vi "Main.vi"() -> ()   [LabVIEW 2019]
doc: "This sample project is built upon the standard state machine template and shows how you could create an application that acquires, analyzes, and presents data. It includes functionality for presenting configuration dialogs, preserving settings between executions, loading and saving data, as well as exporting graph images and text files.\n\nIt is most appropriate for data that is acquired instantly as it does not allow for screen updates mid acquisition nor does it allow for continuous streaming to disk."
uses:
  controls/State.ctl
  controls/Data.ctl
  controls/UI References.ctl
  controls/Graph Data.ctl
  <vilib>/Utility/miscctls.llb/LVAnnotationListTypeDef.ctl
  <vilib>/Utility/miscctls.llb/LVCursorListTypeDef.ctl
  controls/User Specified Data.ctl
  controls/HW Configuration.ctl
  controls/Simulated Signal Type.ctl
  controls/Analysis Configuration.ctl
  controls/New Data Behavior.ctl
  subVIs/Settings Dialog.vi
panel:
  in  "Settings":bool
  in  "Snapshot":bool
  in  "Analyze":bool
  in  "Clear":bool
  in  "Exit":bool
  in  "Acquire":bool
  in  "Export":bool
  in  "Save Data":bool
  in  "Load Data":bool
  out "Graph":waveform(dbl)[](graph)
  out "Status Bar":string
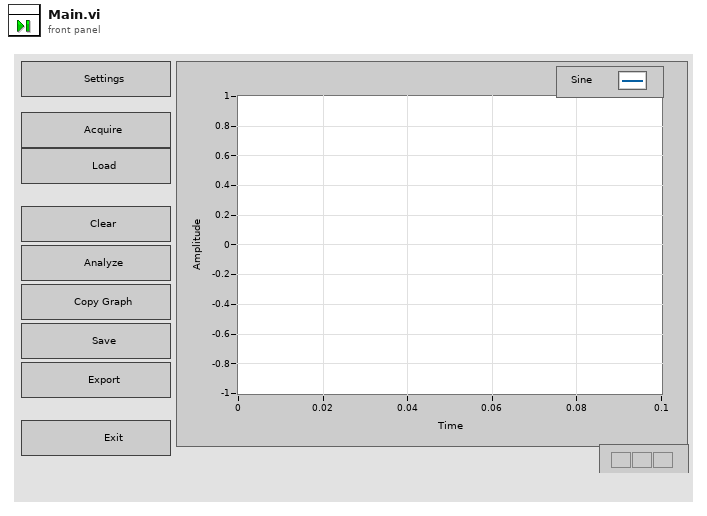
[diagram p1: front panel]
types:
  T1 = typedef "Data.ctl" = cluster{"UI References":T2, "Graph Data":T3, "User Specified":T6}
  T2 = typedef "UI References.ctl" = cluster{"Exit Ref":refnum<vi>, "Save Ref":refnum<vi>, "Open Ref":refnum<vi>, "Export Ref":refnum<vi>, "Acquire Ref":refnum<vi>, "Configure Ref":refnum<vi>, "Graph Ref":refnum<vi>, "Clear Ref":refnum<vi>, "Analyze Ref":refnum<vi>, "Status Ref":refnum<vi>, "Snapshot Ref":refnum<vi>}
  T3 = typedef "Graph Data.ctl" = cluster{"Data":waveform(dbl)[], "Annotation List":T4, "Cursor List":T5, "Analysis Data":waveform(dbl)[]}
  T4 = typedef "LVAnnotationListTypeDef.ctl" = cluster{"Name":string, "Color":u32, "Style":u8, "Point Style":u8, "Name Visible":bool, "Allow Drag":bool, "Annotation Mode":u32, "Plot":i32, "Index":i32, "Position":cluster{"X":dbl, "Y":dbl}, "X Scale":u32, "Y Scale":u32, "Show Arrow":bool, "Lock Name":bool, "Plot Area":i32, "Label Offset":cluster{"X":dbl, "Y":dbl}}[]
  T5 = typedef "LVCursorListTypeDef.ctl" = cluster{"Name":string, "Color":u32, "Style":u8, "Point Style":u8, "Name Visible":bool, "Allow Drag":bool, "Cursor Mode":u32, "Plot":i32, "Index":i32, "Position":cluster{"X":dbl, "Y":dbl}, "X Scale":u32, "Y Scale":u32, "Watch Plots":i32[], "Watch All Plots":bool, "Plot Area":i32, "Label Offset":cluster{"X":dbl, "Y":dbl}}[]
  T6 = typedef "User Specified Data.ctl" = cluster{"Hardware Configuration":T7, "Analysis Configuration":T9, "New Data Behavior":T10}
  T7 = typedef "HW Configuration.ctl" = cluster{"HW Refnum <Replace Me>":string, "Signal Type <Replace Me>":T8}
  T8 = typedef "Simulated Signal Type.ctl" = enum16{"Sine Wave", "Square Wave"}
  T9 = typedef "Analysis Configuration.ctl" = cluster{"Statistics":bool}
  T10 = typedef "New Data Behavior.ctl" = enum16{"Replace", "Overlay", "Append"}
  T11 = typedef "State.ctl" = enum16{"Initialize", "Wait for Event", "Update UI", "Configure", "Acquire", "Load Data", "Save Data", "Clear Data", "Export Data", "Analyze", "Copy Graph", "Exit"}
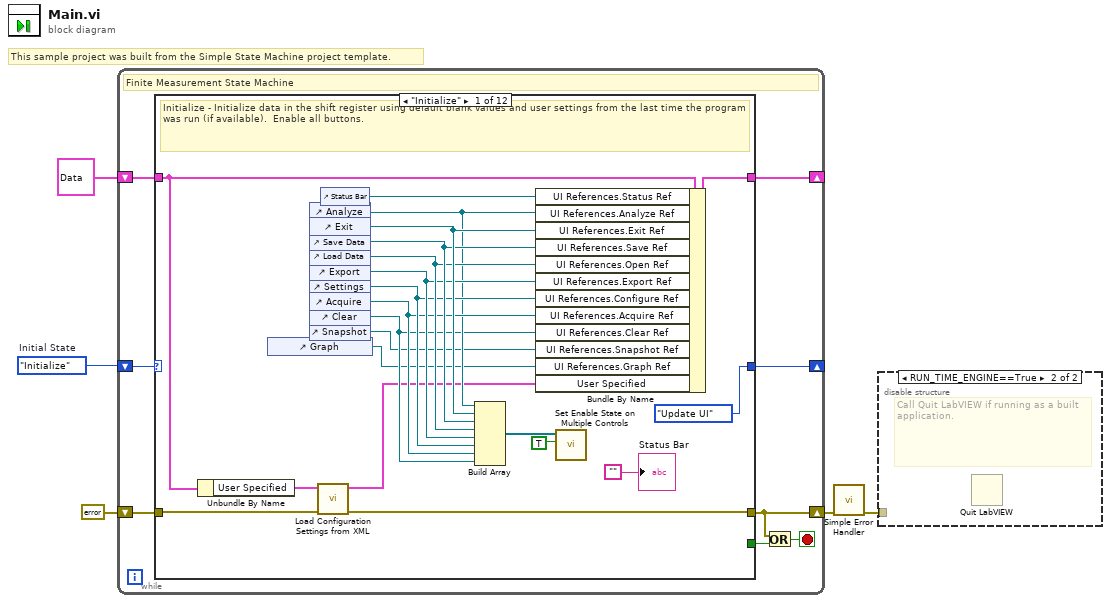
[diagram p0: block diagram]
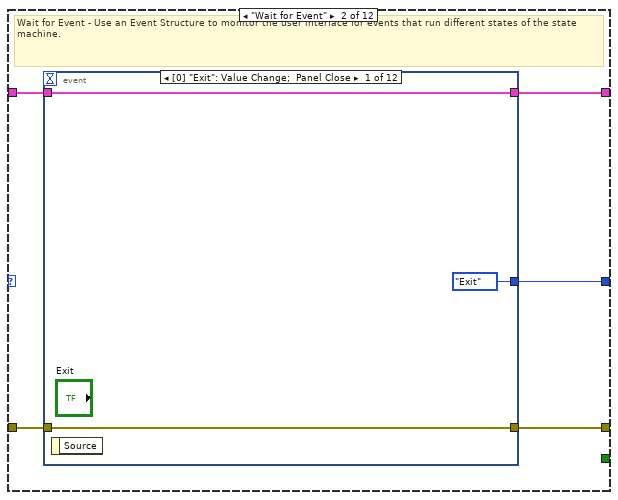
[diagram p3: hidden frame]
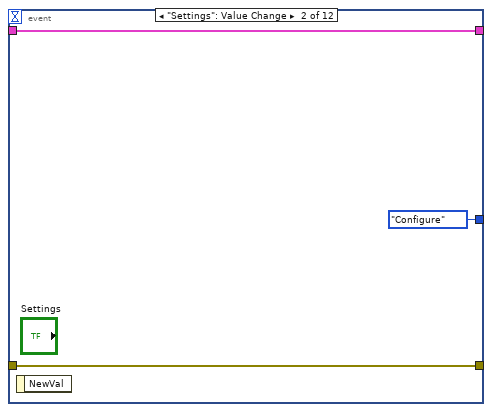
[diagram p4: hidden frame]
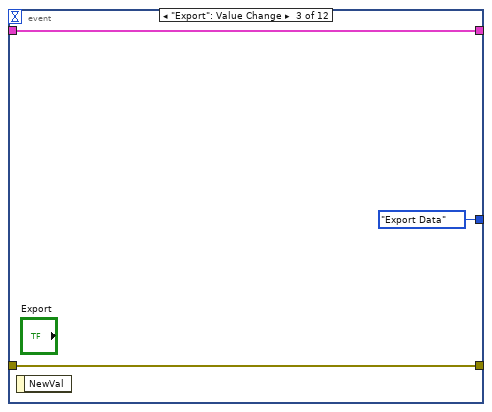
[diagram p5: hidden frame]
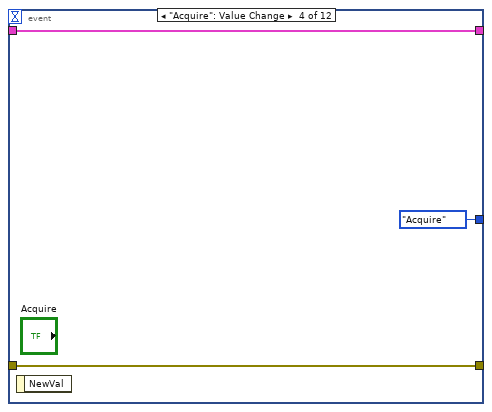
[diagram p6: hidden frame]
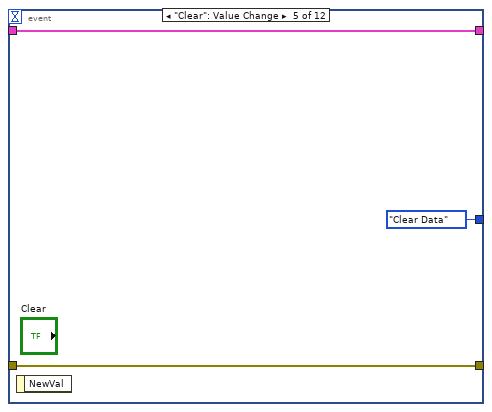
[diagram p7: hidden frame]
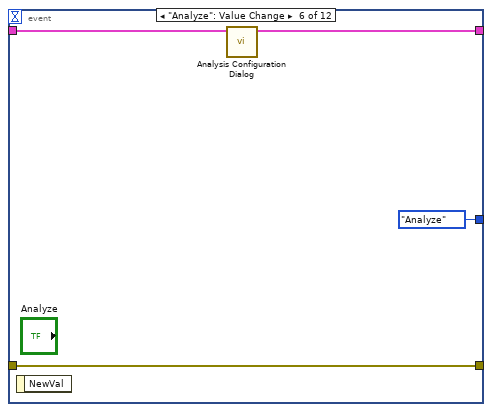
[diagram p8: hidden frame]
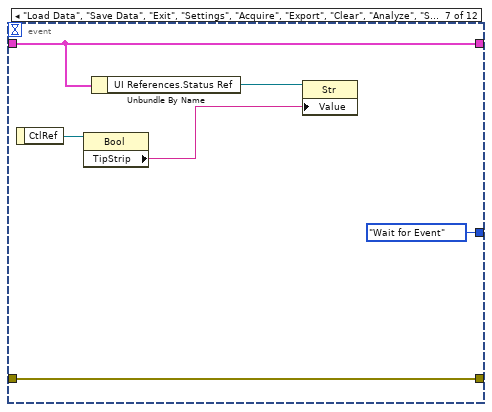
[diagram p9: hidden frame]
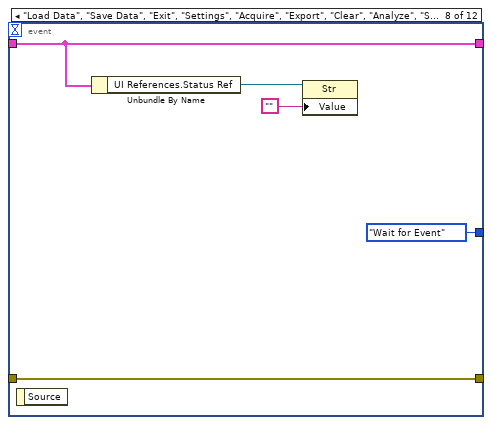
[diagram p10: hidden frame]
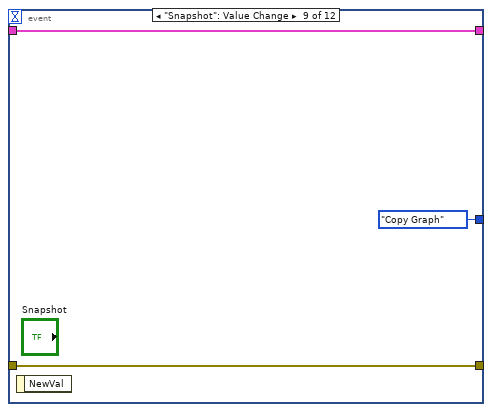
[diagram p11: hidden frame]
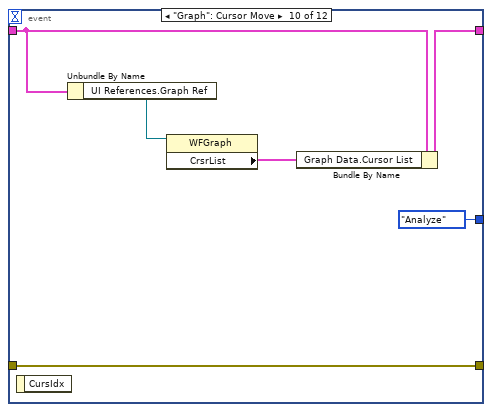
[diagram p12: hidden frame]
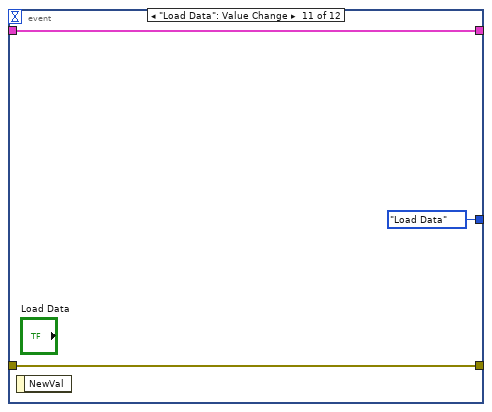
[diagram p13: hidden frame]
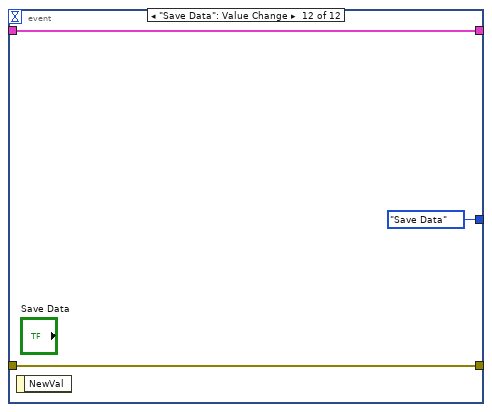
[diagram p14: hidden frame]
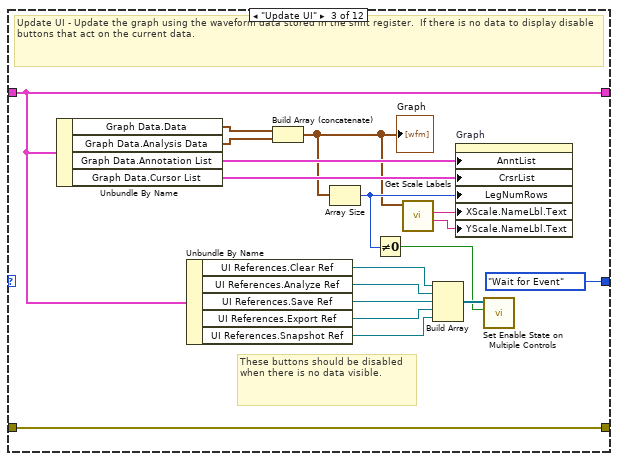
[diagram p15: hidden frame]
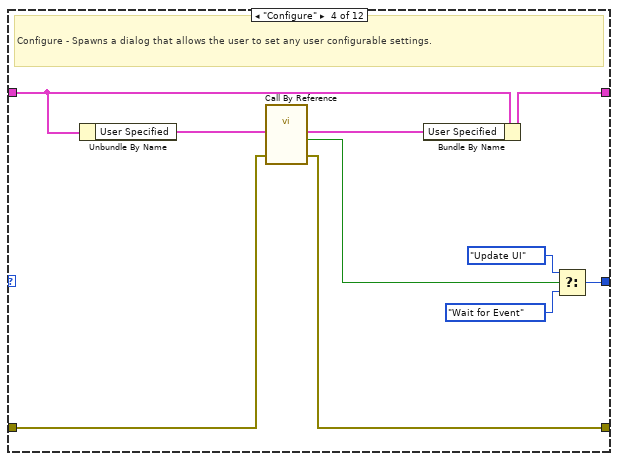
[diagram p16: hidden frame]
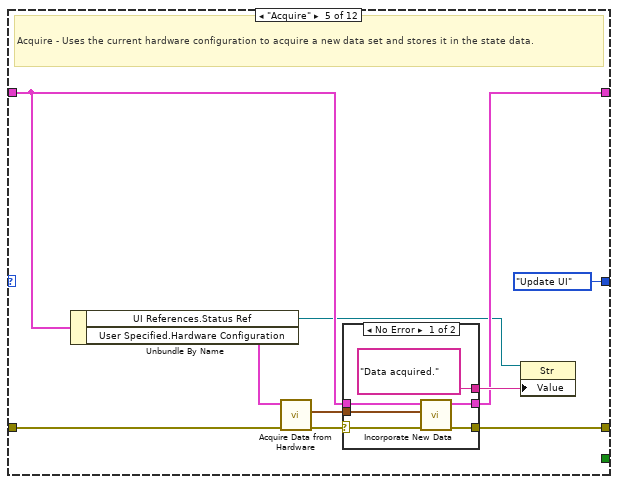
[diagram p17: hidden frame]
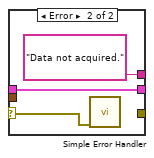
[diagram p18: hidden frame]
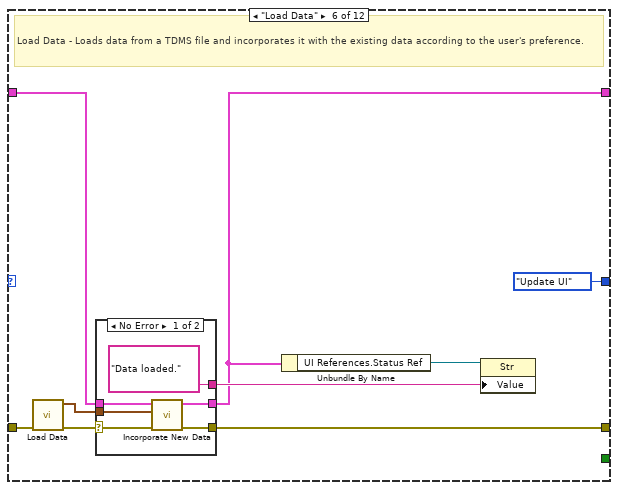
[diagram p19: hidden frame]
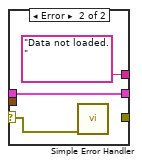
[diagram p20: hidden frame]
diagram:
  w5 = State."Initialize"  # Initial State
  # "This sample project was built from the Simple State Machine project template."
  n1 = while {
    shift-right: [w12] -> _
    shift-left: w5 -> [w13]
    shift-right: [w10] -> _
    shift-left: T1 {"UI References"={"Exit Ref"=refnum, "Save Ref"=refnum, "Open Ref"=refnum, "Export Ref"=refnum, "Acquire Ref"=refnum, "Configure Ref"=refnum, "Graph Ref"=refnum, "Clear Ref"=refnum, "Analyze Ref"=refnum, "Status Ref"=refnum, "Snapshot Ref"=refnum}, "Graph Data"={"Data"=[], "Annotation List"=[], "Cursor List"=[], "Analysis Data"=[]}, "User Specified"={"Hardware Configuration"={"HW Refnum <Replace Me>"="", "Signal Type <Replace Me>"=enum."Sine Wave"}, "Analysis Configuration"={"Statistics"=TRUE}, "New Data Behavior"=enum."Replace"}} ("Data") -> [w11]
    shift-right: [w6] -> w3
    shift-left: errorcluster {"status"=FALSE, "code"=0, "source"=""} ("error constant") -> [w9]
    stop <- w7 stop-if-true
    # "Finite Measurement State Machine"
    n2 = case shown="\"Initialize\"" w13 {
      tunnel: [State."Update UI" ("Next State") w39 State."Wait for Event" ("(Value Not Used)") w106 State."Update UI" ("Next State") State."Update UI" ("(Value Not Used)") State."Wait for Event" ("(Value Not Used)") State."Wait for Event" ("(Value Not Used)") State."Update UI" ("(Value Not Used)") State."Update UI" ("(Value Not Used)") State."Wait for Event" ("(Value Not Used)") w194] -> w12
      tunnel: [_ _ _ _ _ _ _ _ _ _ _ w193] -> w8
      tunnel: w11 -> [w25 w38 w99 w112 w118 w140 w153 w165 w176 w179 w185 w191]
      tunnel: [w33 w37 w99 w111 w117 w134 w153 w165 w175 w179 w185 w191] -> w10
      tunnel: w9 -> [w23 w36 w102 w110 w120 w139 w155 w168 w178 w180 w184 w188]
      tunnel: [w22 w35 w102 w109 w113 w138 w151 w162 w178 w180 w183 w187] -> w6
      frame "Initialize" {
        # "Initialize - Initialize data in the shift register using default blank values and user settings from the last time the program was run (if available).  Enable all buttons."
        n3 = Unbundle By Name(w25) -> ("User Specified"=w24:T6)
        n4 = control-ref of="Graph"() -> (w14:refnum<vi>)
        n5 = control-ref of="Analyze"() -> (w21:refnum<vi>)
        n6 = control-ref of="Exit"() -> (w32:refnum<vi>)
        n7 = control-ref of="Save Data"() -> (w31:refnum<vi>)
        n8 = control-ref of="Load Data"() -> (w30:refnum<vi>)
        n9 = control-ref of="Export"() -> (w29:refnum<vi>)
        n10 = control-ref of="Settings"() -> (w28:refnum<vi>)
        n11 = control-ref of="Acquire"() -> (w27:refnum<vi>)
        n12 = control-ref of="Clear"() -> (w19:refnum<vi>)
        n13 = control-ref of="Snapshot"() -> (w15:refnum<vi>)
        n14 = call "Load Configuration Settings from XML.vi"("error in (no error)"=w23, "User Configuration in"=w24) -> ("error out"=w22:errorcluster, "User Configuration out"=w17:T6)  [unwired: 8 in]
        n15 = control-ref of="Status Bar"() -> (w20:refnum<vi>)
        n16 = Build Array(w21, w32, w31, w30, w29, w28, w27, w19) -> (w26:refnum<vi>[])
        n17 = Bundle By Name(cluster=w25, "UI References.Status Ref"=w20, "UI References.Analyze Ref"=w21, "UI References.Exit Ref"=w32, "UI References.Save Ref"=w31, "UI References.Open Ref"=w30, "UI References.Export Ref"=w29, "UI References.Configure Ref"=w28, "UI References.Acquire Ref"=w27, "UI References.Clear Ref"=w19, "UI References.Snapshot Ref"=w15, "UI References.Graph Ref"=w14, "User Specified"=w17) -> (w33:T1)
        n18 = call "Set Enable State on Multiple Controls.vi"("Enable?"=TRUE, "Controls"=w26) -> ()  [unwired: 10 in]
        "Status Bar" <- "" ("Status Bar")
      }
      frame "Wait for Event" {
        # "Wait for Event - Use an Event Structure to monitor the user interface for events that run different states of the state machine."
        n19 = event shown="[0] \"Exit\": Value Change;  Panel Close" {
          selector: _ -> [_ _ _ _ _ _ _ _ _ _ _ _]
          dyn-events: _ -> [_ _ _ _ _ _ _ _ _ _ _ _]
          timeout: _ -> [_ _ _ _ _ _ _ _ _ _ _ _]
          tunnel: [State."Exit" ("Next State") State."Configure" ("Next State") State."Export Data" ("Next State") State."Acquire" ("Next State") State."Clear Data" ("Next State") State."Analyze" ("Next State") State."Wait for Event" ("Next State") State."Wait for Event" ("Next State") State."Copy Graph" ("Next State") State."Analyze" ("Next State") State."Load Data" ("Next State") State."Save Data" ("Next State")] -> w39
          tunnel: w38 -> [w41 w45 w48 w51 w54 w56 w62 w68 w72 w73 w80 w83]
          tunnel: [w41 w45 w48 w51 w54 w55 w62 w68 w72 w76 w80 w83] -> w37
          tunnel: w36 -> [w40 w44 w47 w50 w53 w58 w64 w69 w71 w78 w79 w82]
          tunnel: [w40 w44 w47 w50 w53 w58 w64 w69 w71 w78 w79 w82] -> w35
          event "Exit": Value Change; Panel Close {
            n20 = event-data() -> ()  [unwired: 1 in, 1 out]
          }
          event "Settings": Value Change {
            n21 = event-data() -> ()  [unwired: 1 in, 1 out]
          }
          event "Export": Value Change {
            n22 = event-data() -> ()  [unwired: 1 in, 1 out]
          }
          event "Acquire": Value Change {
            n23 = event-data() -> ()  [unwired: 1 in, 1 out]
          }
          event "Clear": Value Change {
            n24 = event-data() -> ()  [unwired: 1 in, 1 out]
          }
          event "Analyze": Value Change {
            n25 = event-data() -> ()  [unwired: 1 in, 1 out]
            n26 = call "Analysis Configuration Dialog.vi"("Data in"=w56) -> ("Data out"=w55:T1)  [unwired: 10 in]
          }
          event "Load Data", "Save Data", "Exit", "Settings", "Acquire", "Export", "Clear", "Analyze", "Snapshot": Mouse Enter {
            n27 = event-data() -> ("CtlRef"=w63:refnum<vi>)  [unwired: 1 in]
            n28 = property class="Bool"(reference=w63) -> ("TipStrip"=w60:string)  [unwired: 1 in, 2 out]
            n29 = Unbundle By Name(w62) -> ("UI References.Status Ref"=w61:refnum<vi>)
            n30 = property class="Str"(reference=w61, "Value"=w60) -> ()  [unwired: 1 in, 2 out]
          }
          event "Load Data", "Save Data", "Exit", "Settings", "Acquire", "Export", "Clear", "Analyze", "Snapshot": Mouse Leave {
            n31 = event-data() -> ()  [unwired: 1 in, 1 out]
            n32 = Unbundle By Name(w68) -> ("UI References.Status Ref"=w67:refnum<vi>)
            n33 = property class="Str"(reference=w67, "Value"="") -> ()  [unwired: 1 in, 2 out]
          }
          event "Snapshot": Value Change {
            n34 = event-data() -> ()  [unwired: 1 in, 1 out]
          }
          event "Graph": Cursor Move {
            n35 = event-data() -> ()  [unwired: 1 in, 1 out]
            n36 = Unbundle By Name(w73) -> ("UI References.Graph Ref"=w75:refnum<vi>)
            n37 = property class="WFGraph"(reference=w75) -> ("CrsrList"=w74:T5)  [unwired: 1 in, 2 out]
            n38 = Bundle By Name(cluster=w73, "Graph Data.Cursor List"=w74) -> (w76:T1)
          }
          event "Load Data": Value Change {
            n39 = event-data() -> ()  [unwired: 1 in, 1 out]
          }
          event "Save Data": Value Change {
            n40 = event-data() -> ()  [unwired: 1 in, 1 out]
          }
        }
      }
      frame "Update UI" {
        # "These buttons should be disabled when there is no data visible."
        # "Update UI - Update the graph using the waveform data stored in the shift register.  If there is no data to display disable buttons that act on the current data."
        n41 = Unbundle By Name(w99) -> ("Graph Data.Data"=w95:waveform(dbl)[], "Graph Data.Analysis Data"=w85:waveform(dbl)[], "Graph Data.Annotation List"=w100:T4, "Graph Data.Cursor List"=w96:T5)
        n42 = Unbundle By Name(w99) -> ("UI References.Clear Ref"=w91:refnum<vi>, "UI References.Analyze Ref"=w90:refnum<vi>, "UI References.Save Ref"=w98:refnum<vi>, "UI References.Export Ref"=w88:refnum<vi>, "UI References.Snapshot Ref"=w89:refnum<vi>)
        n43 = Build Array (concatenate)(w95, w85) -> (w93:waveform(dbl)[])
        "Graph" <- w93
        n44 = Array Size(array=w93) -> (size(s)=w94:i32)
        n45 = Not Equal To 0?(x=w94) -> (x != 0?=w92:bool)
        n46 = call "Get Scale Labels.vi"("Array of Waveforms"=w93) -> ("Y Scale Label Text"=w86:string, "X Scale Label Text"=w87:string)  [unwired: 9 in]
        n47 = Build Array(w91, w90, w98, w88, w89) -> (w97:refnum<vi>[])
        n48 = property on="Graph" class="WFGraph (strict)"("AnntList"=w100, "CrsrList"=w96, "LegNumRows"=w94, "XScale.NameLbl.Text"=w87, "YScale.NameLbl.Text"=w86) -> ()  [unwired: 2 in, 2 out]
        n49 = call "Set Enable State on Multiple Controls.vi"("Enable?"=w92, "Controls"=w97) -> ()  [unwired: 10 in]
      }
      frame "Configure" {
        # "Configure - Spawns a dialog that allows the user to set any user configurable settings."
        n50 = Unbundle By Name(w112) -> ("User Specified"=w104:T6)
        n51 = call-by-ref "?"("error in (no error)"=w110, "Configuration in"=w104) -> ("error out"=w109:errorcluster, "UI Refresh Needed?"=w108:bool, "Configuration out"=w103:T6)  [unwired: 9 in, 2 out]
        n52 = Bundle By Name(cluster=w112, "User Specified"=w103) -> (w111:T1)
        n53 = Select(t=State."Update UI" ("Next State if true"), s=w108, f=State."Wait for Event" ("Next State if false")) -> (s? t:f=w106:T11)
      }
      frame "Acquire" {
        # "Acquire - Uses the current hardware configuration to acquire a new data set and stores it in the state data."
        n54 = Unbundle By Name(w118) -> ("UI References.Status Ref"=w114:refnum<vi>, "User Specified.Hardware Configuration"=w121:T7)
        n55 = call "Acquire Data from Hardware.vi"("error in (no error)"=w120, "Hardware Configuration"=w121) -> ("error out"=w115:errorcluster, "Graph Data"=w116:waveform(dbl)[])  [unwired: 8 in]
        n56 = case shown="No Error" w115 {
          selector: w115 -> [w125 w130]
          tunnel: w118 -> [w124 w131]
          tunnel: [w128 w131] -> w117
          tunnel: [w127 _] -> w113
          tunnel: w116 -> [w126 _]
          tunnel: ["Data acquired." ("Data acquired") "Data not acquired." ("Data not acquired")] -> w119
          frame No Error {
            n57 = call "Incorporate New Data.vi"("error in (no error)"=w125, "New Graph Data"=w126, "Data in"=w124) -> ("error out"=w127:errorcluster, "Data out"=w128:T1)  [unwired: 7 in]
          }
          frame Error {
            n58 = call <vilib>:"Simple Error Handler.vi"("error in (no error)"=w130) -> ()  [unwired: 4 in, 5 out]
          }
        }
        n59 = property class="Str"(reference=w114, "Value"=w119) -> ()  [unwired: 1 in, 2 out]
      }
      frame "Load Data" {
        # "Load Data - Loads data from a TDMS file and incorporates it with the existing data according to the user's preference."
        n60 = call "Load Data.vi"("error in (no error)"=w139) -> ("error out"=w136:errorcluster, "New Graph Data"=w133:waveform(dbl)[])  [unwired: 9 in]
        n61 = case shown="No Error" w136 {
          selector: w136 -> [w143 w148]
          tunnel: w140 -> [w142 w149]
          tunnel: [w146 w149] -> w134
          tunnel: [w145 _] -> w138
          tunnel: w133 -> [w144 _]
          tunnel: ["Data loaded." ("Data loaded") "Data not loaded." ("Data not loaded")] -> w135
          frame No Error {
            n62 = call "Incorporate New Data.vi"("error in (no error)"=w143, "New Graph Data"=w144, "Data in"=w142) -> ("error out"=w145:errorcluster, "Data out"=w146:T1)  [unwired: 7 in]
          }
          frame Error {
            n63 = call <vilib>:"Simple Error Handler.vi"("error in (no error)"=w148) -> ()  [unwired: 4 in, 5 out]
          }
        }
        n64 = Unbundle By Name(w134) -> ("UI References.Status Ref"=w132:refnum<vi>)
        n65 = property class="Str"(reference=w132, "Value"=w135) -> ()  [unwired: 1 in, 2 out]
      }
      frame "Save Data" {
        # "Save Data - Saves the existing measurement data to a TDMS file."
        n66 = Unbundle By Name(w153) -> ("UI References.Status Ref"=w152:refnum<vi>, "Graph Data.Data"=w156:waveform(dbl)[])
        n67 = call "Save Data.vi"("error in (no error)"=w155, "Data"=w156) -> ("error out"=w154:errorcluster)  [unwired: 9 in]
        n68 = case shown="No Error" w154 {
          selector: w154 -> [w158 w161]
          tunnel: ["Data saved." ("Data saved") "Data not saved." ("Data not saved")] -> w150
          tunnel: [w158 _] -> w151
          frame No Error {
          }
          frame Error {
            n69 = call <vilib>:"Simple Error Handler.vi"("error in (no error)"=w161) -> ()  [unwired: 4 in, 5 out]
          }
        }
        n70 = property class="Str"(reference=w152, "Value"=w150) -> ()  [unwired: 1 in, 2 out]
      }
      frame "Export Data" {
        # "Export Data - Exports the currently loaded measurement and analysis data to a text file that can be imported into a spreadsheet or other application."
        n71 = Unbundle By Name(w165) -> ("UI References.Status Ref"=w163:refnum<vi>, "Graph Data"=w164:T3)
        n72 = call "Export Data.vi"("error in (no error)"=w168, "Graph Data"=w164) -> ("error out"=w166:errorcluster)  [unwired: 9 in]
        n73 = case shown="No Error" w166 {
          selector: w166 -> [w170 w173]
          tunnel: ["Data exported." ("Data exported") "Data not exported." ("Data not exported")] -> w167
          tunnel: [w170 _] -> w162
          frame No Error {
          }
          frame Error {
            n74 = call <vilib>:"Simple Error Handler.vi"("error in (no error)"=w173) -> ()  [unwired: 4 in, 5 out]
          }
        }
        n75 = property class="Str"(reference=w163, "Value"=w167) -> ()  [unwired: 1 in, 2 out]
      }
      frame "Clear Data" {
        # "Clear Data - Clears the data currently in the graph."
        n76 = Bundle By Name(cluster=w176, "Graph Data"=T3 {"Data"=[], "Annotation List"=[], "Cursor List"=[], "Analysis Data"=[]} ("Graph")) -> (w175:T1)
      }
      frame "Analyze" {
        # "#CodeRecommended - Add your own signal analysis here."
        # "Analyze - Analyzes the measurement data."
        n77 = Unbundle By Name(w179) -> ("Graph Data"=w181:T3)
        n78 = call "Statistical Analysis.vi"("Graph Data In"=w181) -> ()  [unwired: 9 in, 2 out]
      }
      frame "Copy Graph" {
        # "Copy Graph - Places an image of the graph on the clipboard for pasting into reports or emails."
        n79 = call "Copy Graph to Clipboard.vi"("error in (no error)"=w184, "Graph Data"=w185) -> ("error out"=w183:errorcluster)  [unwired: 9 in]
      }
      frame "Exit" {
        w193 = TRUE  # Stop Loop?
        w194 = State."Exit"  # (Value Not Used)
        # "Exit - Saves the user's settings to an XML file and stops execution."
        n80 = Unbundle By Name(w191) -> ("UI References.Status Ref"=w189:refnum<vi>, "User Specified"=w192:T6)
        n81 = call "Save Configuration Settings to XML.vi"("error in (no error)"=w188, "User Configuration"=w192) -> ("error out"=w187:errorcluster)  [unwired: 9 in]
        n82 = property class="Str"(reference=w189, "Value"="Application exit." ("Stopped")) -> ()  [unwired: 1 in, 2 out]
      }
    }
    n83 = Or(x=w6, y=w8) -> (x .or. y?=w7:bool)
  }
  n84 = call <vilib>:"Simple Error Handler.vi"("error in (no error)"=w3) -> ("error out"=w1:errorcluster)  [unwired: 4 in, 4 out]
  n85 = disable-structure shown="RUN_TIME_ENGINE==True" {
    disable-tunnel: w1 -> [_ _]
    frame condition #0 (active) {
    }
    frame condition #1 {
      # "Call Quit LabVIEW if running as a built application."
      n86 = Quit LabVIEW() -> ()  [unwired: 1 in]
    }
  }
